vi "Gen - Popup Rename Procedure No Ref.vi"(5 "Current File name":string, 6 "Type":enum16{"Error", "Info"}(ring)=enum."Info", 7 "List of Template":string[](array[string]), 8 "Error in":errorcluster, 9 "Button text":string[](array[string])=["YES", "NO"], 10 "Message in":string, 11 "Header":string) -> (0 "Error out":errorcluster, 2 "procedure no./ref.  filename":string, 3 "Yes?":bool)   [LabVIEW 2020]
uses:
  Control/State - eFGV.ctl
  04f009c0-d03a-4eb7-a55f-4b75b582feef.vi
  <vilib>/Comparison/Equal/Equal Functor/Equal Functor.lvclass
panel:
  in  "Warning":string
  in  "Template Name":string
  out "Type Error":bool
  in  "No":bool
  in  "Yes":bool
  in  "Cancel":bool
  out "Type Info":bool
  in  "OK":bool
  out "Header out":string
  in  "Exit":bool
  out "Message":string
  in  "Auto Close?":bool
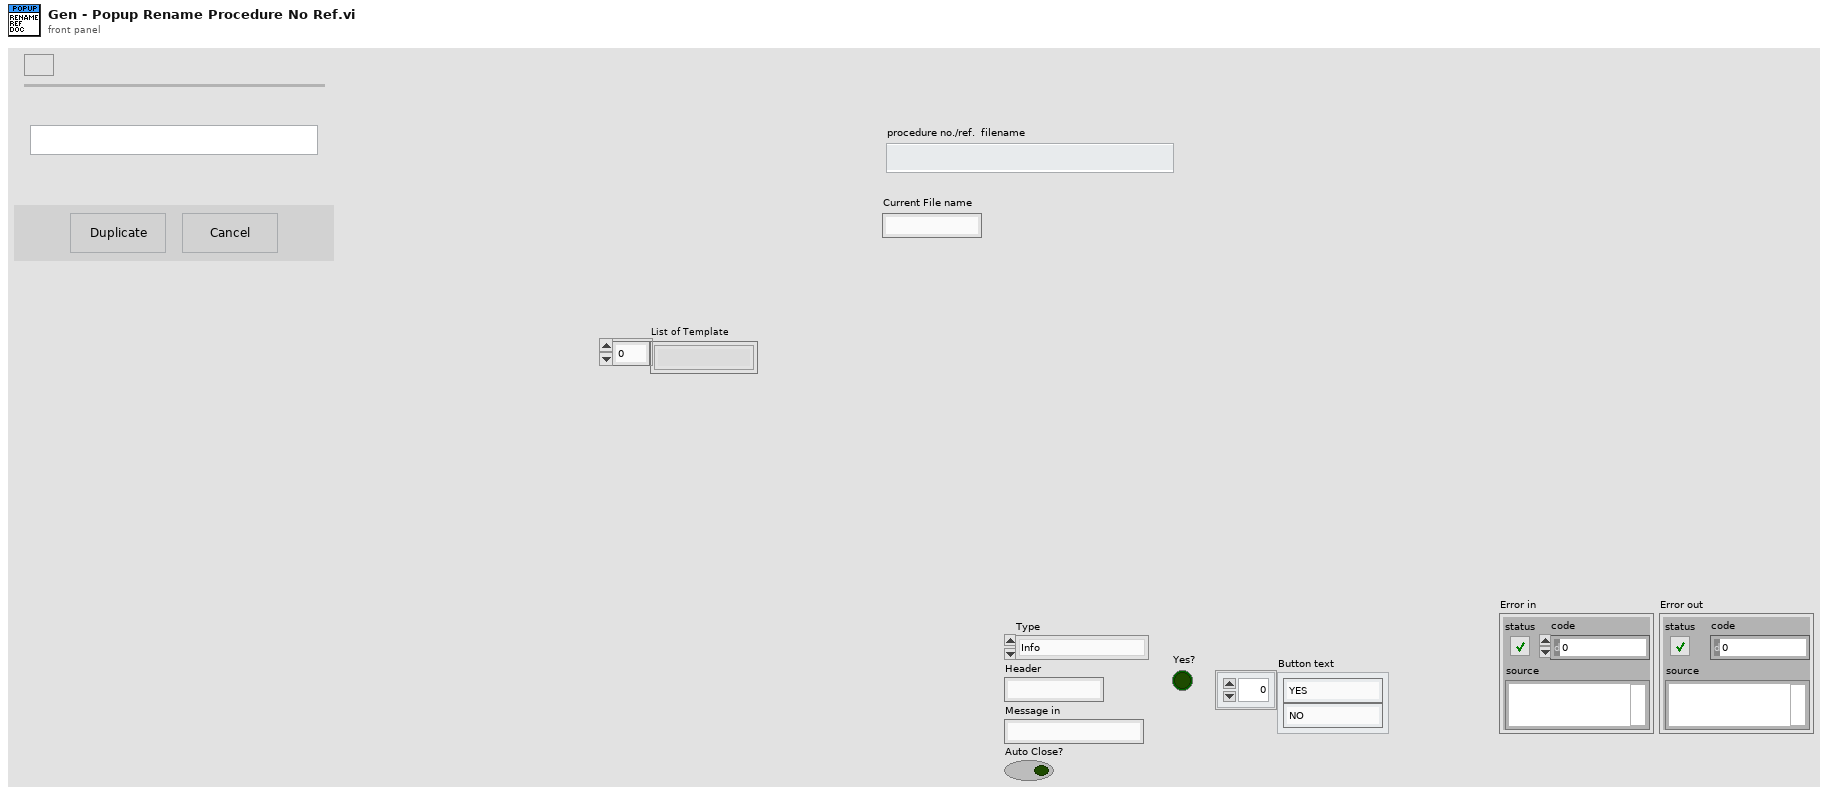
[diagram p1: front panel]
types:
  T1 = typedef "State - eFGV.ctl" = enum16{"Init", "Read", "Write", "Exit"}
  T2 = enum32{"Invalid", "Default", "Floating", "Floating/Auto-Hide", "Modal"}
  T3 = enum8{"Enabled", "Disabled", "Disabled and Grayed Out"}
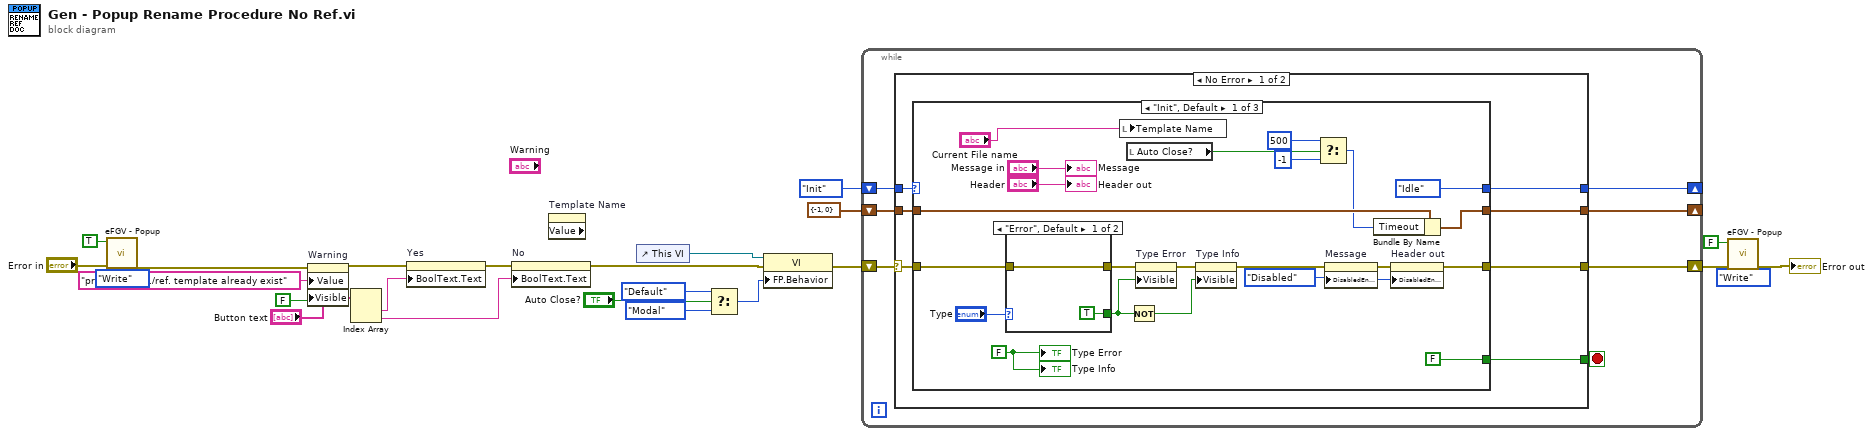
[diagram p0: block diagram]
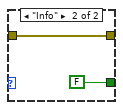
[diagram p2: hidden frame]
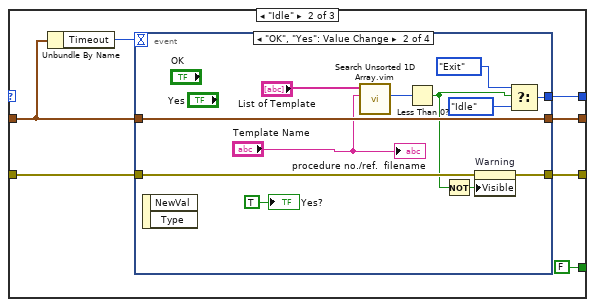
[diagram p3: hidden frame]
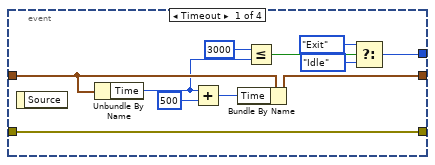
[diagram p4: hidden frame]
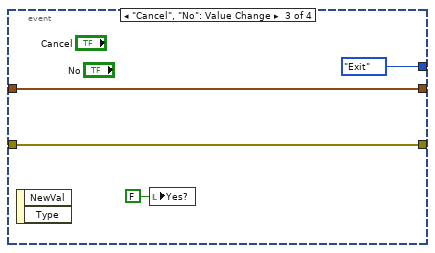
[diagram p5: hidden frame]
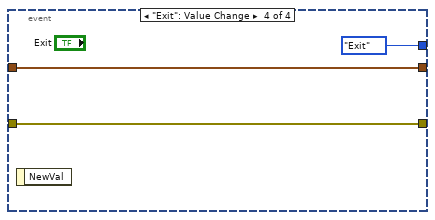
[diagram p6: hidden frame]
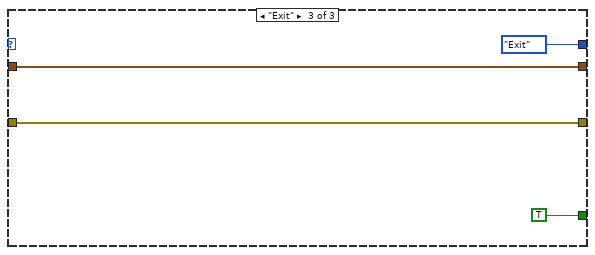
[diagram p7: hidden frame]
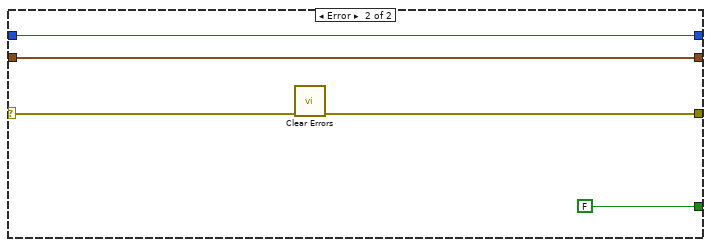
[diagram p8: hidden frame]
diagram:
  n1 = call "eFGV - Popup.vi"("Action"=State_-_eFGV."Write", "Error In"="Error in", "Popup"=TRUE) -> ("Error Out"=w3:errorcluster)  [unwired: 6 in, 2 out]
  n2 = property on="Warning" class="Str"(error in=w3, "Value"="procedure no./ref. template already exist" ("Warning"), "Visible"=FALSE) -> (error out=w4:errorcluster)  [unwired: 1 in, 1 out]
  n3 = Index Array(array="Button text") -> (element #1=w13:string, element #2=w12:string)  [unwired: 2 in]
  n4 = property on="Yes" class="Bool"(error in=w4, "BoolText.Text"=w13) -> (error out=w16:errorcluster)  [unwired: 1 in, 1 out]
  n5 = property on="No" class="Bool"(error in=w16, "BoolText.Text"=w12) -> (error out=w15:errorcluster)  [unwired: 1 in, 1 out]
  n6 = property on="Template Name" class="Str" props=["Value"]() -> ()  [unwired: 2 in, 3 out]
  n7 = control-ref of="This VI"() -> (w22:refnum<vi>)
  n8 = Select(t=T2."Default" ("Front Panel Window:Behavior"), s="Auto Close?", f=T2."Modal") -> (s? t:f=w18:T2)
  n9 = property class="VI"(reference=w22, error in=w15, "FP.Behavior"=w18) -> (error out=w21:errorcluster)  [unwired: 1 out]
  n10 = while {
    shift-right: [w29] -> _
    shift-left: enum16{"Init", "Idle", "Exit"}."Init" -> [w30]
    shift-right: [w28] -> w8
    shift-left: w21 -> [w31]
    shift-right: [w25] -> _
    shift-left: cluster{"Timeout":i32, "Time":i32} {"Timeout"=-1, "Time"=0} -> [w26]
    stop <- w27 stop-if-true
    n11 = case shown="No Error" w31 {
      selector: w31 -> [w35 w109]
      tunnel: w30 -> [w38 w110]
      tunnel: [w37 w110] -> w29
      tunnel: [w36 w107] -> w28
      tunnel: [w34 FALSE] -> w27
      tunnel: w26 -> [w33 w106]
      tunnel: [w32 w106] -> w25
      frame No Error {
        n12 = case shown="\"Init\", Default" w38 {
          tunnel: [enum16{"Init", "Idle", "Exit"}."Idle" w71 enum16{"Init", "Idle", "Exit"}."Exit"] -> w37
          tunnel: [w45 w70 w105] -> w36
          tunnel: w35 -> [w52 w69 w105]
          tunnel: [FALSE FALSE TRUE] -> w34
          tunnel: w33 -> [w56 w66 w102]
          tunnel: [w55 w67 w102] -> w32
          frame "Init", Default {
            w48 = T3."Disabled" ("Disabled")
            w40 = FALSE ("Type Error")
            n13 = case shown="\"Error\", Default" "Type" {
              tunnel: [w61 w64] -> w53
              tunnel: w52 -> [w61 w64]
              tunnel: [TRUE FALSE] -> w50
              frame "Error", Default {
              }
              frame "Info" {
              }
            }
            n14 = local write "Template Name"("Current File name") -> ()
            n15 = local read "Auto Close?"() -> (w41:bool)
            n16 = Not(x=w50) -> (.not. x?=w49:bool)
            n17 = property on="Type Error" class="Bool"(error in=w53, "Visible"=w50) -> (error out=w54:errorcluster)  [unwired: 1 in, 1 out]
            n18 = property on="Type Info" class="Bool (strict)"(error in=w54, "Visible"=w49) -> (error out=w46:errorcluster)  [unwired: 1 in, 1 out]
            n19 = Select(t=500 ("Timeout"), s=w41, f=-1 ("Timeout")) -> (s? t:f=w43:i32)
            n20 = property on="Message" class="Str"(error in=w46, "DisabledEnum"=w48) -> (error out=w47:errorcluster)  [unwired: 1 in, 1 out]
            n21 = Bundle By Name(cluster=w56, "Timeout"=w43) -> (w55:cluster{"Timeout":i32, "Time":i32})
            n22 = property on="Header out" class="Str"(error in=w47, "DisabledEnum"=w48) -> (error out=w45:errorcluster)  [unwired: 1 in, 1 out]
            "Message" <- "Message in"
            "Header out" <- "Header"
            "Type Info" <- w40
            "Type Error" <- w40
          }
          frame "Idle" {
            n23 = Unbundle By Name(w66) -> ("Timeout"=w65:i32)
            n24 = event shown="[1] \"OK\", \"Yes\": Value Change" {
              selector: _ -> [_ _ _ _]
              dyn-events: _ -> [_ _ _ _]
              timeout: w65 -> [_ _ _ _]
              tunnel: [w74 w90 enum16{"Init", "Idle", "Exit"}."Exit" enum16{"Init", "Idle", "Exit"}."Exit"] -> w71
              tunnel: [w82 w85 w96 w99] -> w70
              tunnel: w69 -> [w82 w86 w96 w99]
              tunnel: [w80 w94 w97 w100] -> w67
              tunnel: w66 -> [w81 w94 w97 w100]
              event Timeout {
                n25 = event-data() -> ()  [unwired: 1 in, 1 out]
                n26 = Unbundle By Name(w81) -> ("Time"=w77:i32)
                n27 = Add(x=w77, y=500) -> (x+y=w79:i32)
                n28 = Bundle By Name(cluster=w81, "Time"=w79) -> (w80:cluster{"Timeout":i32, "Time":i32})
                n29 = Less Or Equal?(x=3000, y=w77) -> (x <= y?=w75:bool)
                n30 = Select(t=enum16{"Init", "Idle", "Exit"}."Exit", s=w75, f=enum16{"Init", "Idle", "Exit"}."Idle") -> (s? t:f=w74:enum16{"Init", "Idle", "Exit"})
              }
              event "OK", "Yes": Value Change {
                n31 = event-data() -> ()  [unwired: 1 in, 2 out]
                n32 = call "Search Unsorted 1D Array.vim"("element"="Template Name", "unsorted 1D array"="List of Template") -> ("index of element"=w88:i32)  [unwired: 9 in]
                n33 = Less Than 0?(x=w88) -> (x < 0?=w84:bool)
                n34 = Not(x=w84) -> (.not. x?=w83:bool)
                n35 = property on="Warning" class="Str"(error in=w86, "Visible"=w83) -> (error out=w85:errorcluster)  [unwired: 1 in, 1 out]
                n36 = Select(t=enum16{"Init", "Idle", "Exit"}."Exit", s=w84, f=enum16{"Init", "Idle", "Exit"}."Idle") -> (s? t:f=w90:enum16{"Init", "Idle", "Exit"})
                "Yes?" <- TRUE ("Yes?")
                "procedure no./ref.  filename" <- "Template Name"
              }
              event "Cancel", "No": Value Change {
                n37 = event-data() -> ()  [unwired: 1 in, 2 out]
                n38 = local write "Yes?"(FALSE ("Yes?")) -> ()
              }
              event "Exit": Value Change {
                n39 = event-data() -> ()  [unwired: 1 in, 1 out]
              }
            }
          }
          frame "Exit" {
          }
        }
      }
      frame Error {
        n40 = call <vilib>:"Clear Errors.vi"("error in (no error)"=w109) -> ("error out"=w107:errorcluster)  [unwired: 5 in, 1 out]
      }
    }
  }
  n41 = call "eFGV - Popup.vi"("Action"=State_-_eFGV."Write", "Error In"=w8, "Popup"=FALSE) -> ("Error Out"=→"Error out":errorcluster)  [unwired: 6 in, 2 out]
